vi "3.1-Unit Conversion.vi"(3 "Lidar In":dbl, 4 "Steering In":dbl, 5 "Drive In":dbl) -> (0 "Lidar Out":i32, 1 "Steering Out":i32, 2 "Drive Out":i32)   [LabVIEW 2010]
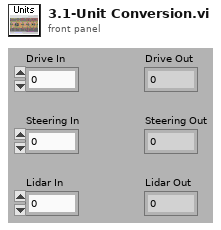
[diagram p1: front panel]
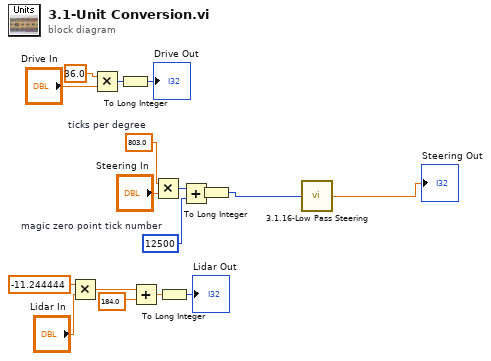
[diagram p0: block diagram]
diagram:
  w14 = 803.0  # ticks per degree
  w12 = 12500  # magic zero point tick number
  n1 = Multiply(x=-11.244444 ("Lidar Scale"), y="Lidar In") -> (x*y=w8:dbl)
  n2 = Multiply(x=36.0, y="Drive In") -> (x*y=w4:i32)
  n3 = To Long Integer(number=w4) -> (32bit integer=→"Drive Out":i32)
  n4 = Add(x=w8, y=184.0 ("Lidar Offset")) -> (x+y=w9:dbl)
  n5 = Multiply(x=w14, y="Steering In") -> (x*y=w13:i32)
  n6 = To Long Integer(number=w9) -> (32bit integer=→"Lidar Out":i32)
  n7 = Add(x=w13, y=w12) -> (x+y=w10:i32)
  n8 = To Long Integer(number=w10) -> (32bit integer=w2:i32)
  n9 = call "3.1.16-Low Pass Steering.vi"("Numeric 2"=w2) -> ("Numeric"=→"Steering Out":dbl)
